vi "HXG2_EXP Valves to Superheat Ctrl.vi"(8 "error in (no error)":errorcluster, 10 "Comp Suct Temp":dbl, 11 "Comp Suct P":dbl) -> (0 "error out":errorcluster, 2 "Multiplier":dbl, 3 "Super Heat (°F)":dbl)   [LabVIEW 2012]
doc: "This VI will calculate the ammount of superheat to the compressor and output a multiplier value that will affect the opening of the EXVs. Output is double 'Superheat' and double 'EXV multiplier'."
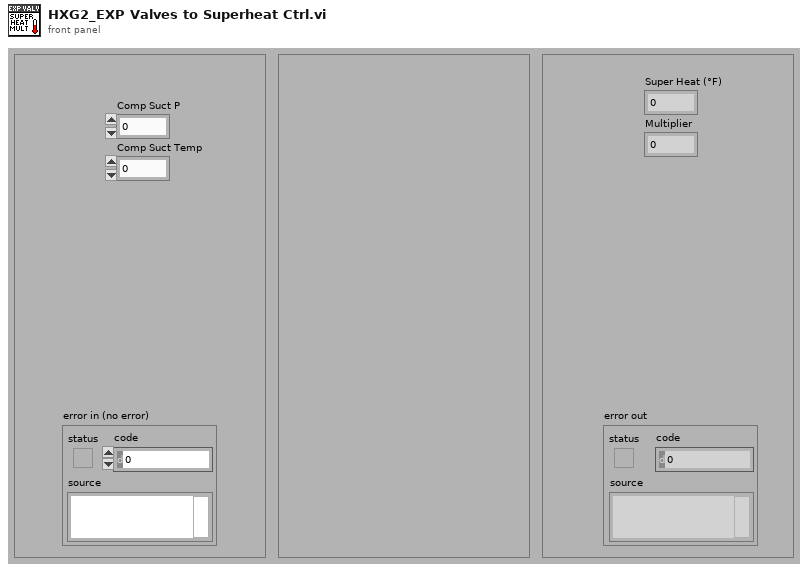
[diagram p1: front panel]
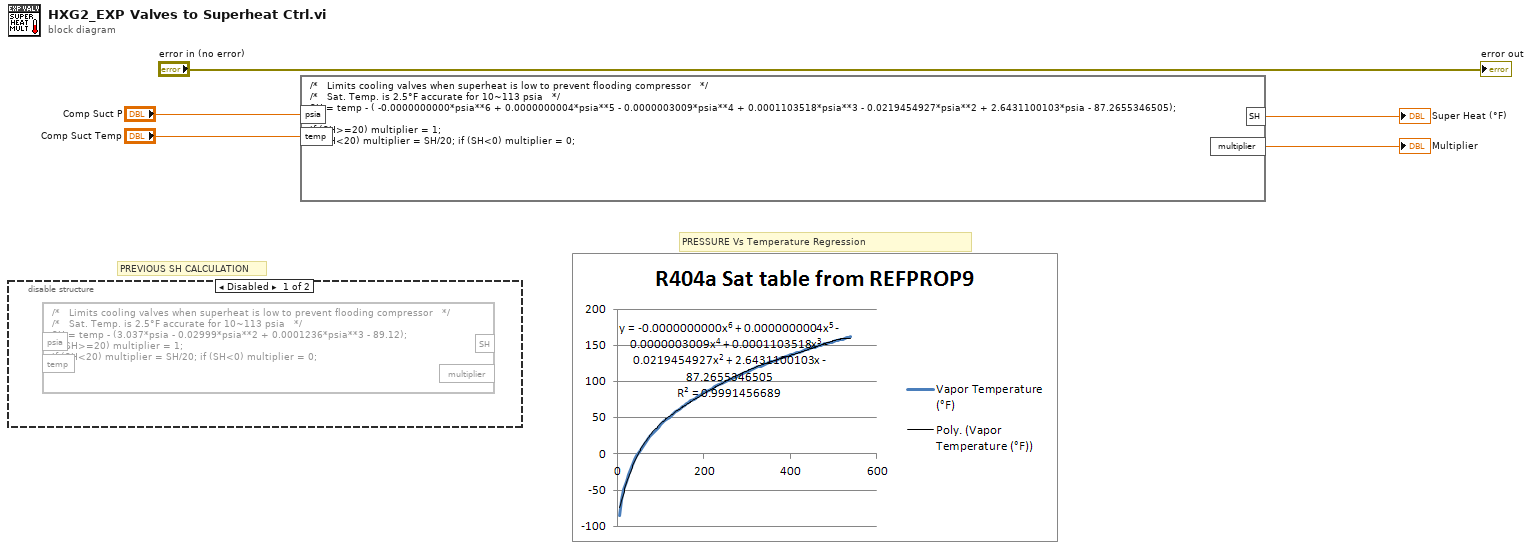
[diagram p0: block diagram]
diagram:
  # "PRESSURE Vs Temperature Regression"
  # "PREVIOUS SH CALCULATION"
  n1 = disable-structure shown="Disabled" {
    frame Disabled {
      n2 = formula code="/*   Limits cooling valves when superheat is low to prevent flooding compressor   */\n/*   Sat. Temp. is 2.5°F accurate for 10~113 psia   */\nSH = temp - (3.037*psia - 0.02999*psia**2 + 0.0001236*psia**3 - 89.12);\nif (SH>=20) multiplier = 1;\nif (SH<20) multiplier = SH/20; if (SH<0) multiplier = 0;"() -> ()  [unwired: 2 in, 2 out]
    }
    frame Enabled {
    }
  }
  n3 = formula code="/*   Limits cooling valves when superheat is low to prevent flooding compressor   */\n/*   Sat. Temp. is 2.5°F accurate for 10~113 psia   */\nSH = temp - ( -0.0000000000*psia**6 + 0.0000000004*psia**5 - 0.0000003009*psia**4 + 0.0001103518*psia**3 - 0.0219454927*psia**2 + 2.6431100103*psia - 87.2655346505);\n\nif (SH>=20) multiplier = 1;\nif (SH<20) multiplier = SH/20; if (SH<0) multiplier = 0;"("psia"="Comp Suct P", "temp"="Comp Suct Temp") -> ("SH"=→"Super Heat (°F)":dbl, "multiplier"=→"Multiplier":dbl)
  "error out" <- "error in (no error)"
